vi "PSVCH_Demo_View.vi"() -> ()   [LabVIEW 2016]
panel:
  in  "Parameter":cluster{"Tag[]":string[], "Time":i64}={"Tag[]"=["VCH1"], "Time"=0}
  out "PData":waveform(dbl)[](graph)=[{"t0"=timestamp(3468473151.3644843 s since 1904-01-01), "dt"=0.001, "Y"=[6.739850074752029e-05, -0.00025439845700241445, -9.34999781361974e-05, -0.00025439845700241445, -0.00025439845700241445, -0.00025439845700241445, -0.0004152969358511465, -0.00025439845700241445, -0.00025439845700241445, 6.739850074752029e-05, -9.34999781361974e-05, -9.34999781361974e-05, -0.0004152969358511465, -9.34999781361974e-05, -0.0004152969358511465, 6.739850074752029e-05, -0.00025439845700241445, -0.00025439845700241445, 6.739850074752029e-05, -0.00025439845700241445, -9.34999781361974e-05, 0.00022829697964875422, -0.00025439845700241445, 0.00022829697964875422, 6.739850074752029e-05, 6.739850074752029e-05, -0.00025439845700241445, -0.00025439845700241445, -0.00025439845700241445, -9.34999781361974e-05, -9.34999781361974e-05, 6.739850074752029e-05, -0.00025439845700241445, -9.34999781361974e-05, -0.0004152969358511465, -0.00025439845700241445, 6.739850074752029e-05, -9.34999781361974e-05, -0.00025439845700241445, -0.00025439845700241445, -9.34999781361974e-05, 6.739850074752029e-05, 6.739850074752029e-05, 6.739850074752029e-05, -0.00025439845700241445, 0.00022829697964875422, -0.00025439845700241445, -0.0004152969358511465, -0.00025439845700241445, -9.34999781361974e-05], "attributes"=variant("NI_ChannelName"=variant(string "1"), "NI_UnitDescription"=variant(string "Volts"))}, {"t0"=timestamp(3468473151.364507 s since 1904-01-01), "dt"=0.001, "Y"=[-0.012665767574885531, -0.012665767574885531, -0.012826630906157108, -0.012826630906157108, -0.012826630906157108, -0.012826630906157108, -0.012504904243597582, -0.012665767574885531, -0.012665767574885531, -0.012665767574885531, -0.0131483575686512, -0.012504904243597582, -0.012665767574885531, -0.012826630906157108, -0.012826630906157108, -0.012826630906157108, -0.012826630906157108, -0.012987494237412326, -0.012665767574885531, -0.012826630906157108, -0.012987494237412326, -0.012504904243597582, -0.012826630906157108, -0.012826630906157108, -0.012826630906157108, -0.012826630906157108, -0.012987494237412326, -0.012665767574885531, -0.012987494237412326, -0.012987494237412326, -0.012826630906157108, -0.012826630906157108, -0.012826630906157108, -0.012826630906157108, -0.012665767574885531, -0.012826630906157108, -0.012826630906157108, -0.012826630906157108, -0.012665767574885531, -0.012504904243597582, -0.012826630906157108, -0.012504904243597582, -0.012987494237412326, -0.012826630906157108, -0.012826630906157108, -0.012826630906157108, -0.012826630906157108, -0.012826630906157108, -0.012826630906157108, -0.012987494237412326], "attributes"=variant("NI_ChannelName"=variant(string "2"), "NI_UnitDescription"=variant(string "Volts"))}, {"t0"=timestamp(3468473151.36453 s since 1904-01-01), "dt"=0.001, "Y"=[0.00011638367757987423, 0.00011638367757987423, 0.00027723671651823503, -4.446936134091291e-05, 0.00011638367757987423, 0.00011638367757987423, -4.446936134091291e-05, 0.0004380897554741851, -4.446936134091291e-05, -0.000205322400244142, -4.446936134091291e-05, 0.00027723671651823503, -4.446936134091291e-05, -4.446936134091291e-05, 0.00027723671651823503, 0.00027723671651823503, -4.446936134091291e-05, -4.446936134091291e-05, 0.00027723671651823503, -4.446936134091291e-05, 0.00027723671651823503, 0.00011638367757987423, -4.446936134091291e-05, 0.0004380897554741851, -4.446936134091291e-05, 0.00011638367757987423, 0.00011638367757987423, 0.00027723671651823503, 0.00011638367757987423, -4.446936134091291e-05, 0.00011638367757987423, 0.00011638367757987423, -4.446936134091291e-05, 0.00011638367757987423, -4.446936134091291e-05, -4.446936134091291e-05, -4.446936134091291e-05, -4.446936134091291e-05, 0.00011638367757987423, 0.00027723671651823503, 0.00011638367757987423, 0.00011638367757987423, -4.446936134091291e-05, 0.00011638367757987423, 0.00011638367757987423, 0.00027723671651823503, 0.00027723671651823503, 0.00027723671651823503, 0.00011638367757987423, -4.446936134091291e-05], "attributes"=variant("NI_ChannelName"=variant(string "3"), "NI_UnitDescription"=variant(string "Volts"))}, {"t0"=timestamp(3468473151.364553 s since 1904-01-01), "dt"=0.001, "Y"=[-0.01584889046687111, -0.01584889046687111, -0.01552708791201146, -0.015687989189449317, -0.015687989189449317, -0.01552708791201146, -0.016009791744276847, -0.015687989189449317, -0.01584889046687111, -0.01584889046687111, -0.01584889046687111, -0.016009791744276847, -0.01584889046687111, -0.016009791744276847, -0.015687989189449317, -0.01584889046687111, -0.016009791744276847, -0.01584889046687111, -0.01584889046687111, -0.015687989189449317, -0.015687989189449317, -0.015687989189449317, -0.01584889046687111, -0.01584889046687111, -0.015687989189449317, -0.01584889046687111, -0.015687989189449317, -0.01584889046687111, -0.01584889046687111, -0.016009791744276847, -0.015687989189449317, -0.01552708791201146, -0.015687989189449317, -0.015687989189449317, -0.01584889046687111, -0.015687989189449317, -0.015687989189449317, -0.015687989189449317, -0.01552708791201146, -0.016009791744276847, -0.015687989189449317, -0.015687989189449317, -0.01536618663455752, -0.01584889046687111, -0.016009791744276847, -0.016170693021666554, -0.015687989189449317, -0.015687989189449317, -0.01552708791201146, -0.01584889046687111], "attributes"=variant("NI_ChannelName"=variant(string "4"), "NI_UnitDescription"=variant(string "Volts"))}, {"t0"=timestamp(3468473151.364576 s since 1904-01-01), "dt"=0.001, "Y"=[0.005178231424439744, 0.005178231424439744, 0.005017342955467275, 0.005178231424439744, 0.005017342955467275, 0.005017342955467275, 0.005017342955467275, 0.005339119893430259, 0.005017342955467275, 0.005178231424439744, 0.005017342955467275, 0.005017342955467275, 0.005178231424439744, 0.005017342955467275, 0.005178231424439744, 0.005017342955467275, 0.005017342955467275, 0.005178231424439744, 0.004856454486512835, 0.005178231424439744, 0.004856454486512835, 0.005178231424439744, 0.005178231424439744, 0.005017342955467275, 0.005178231424439744, 0.005339119893430259, 0.005178231424439744, 0.005339119893430259, 0.005017342955467275, 0.005178231424439744, 0.005017342955467275, 0.005017342955467275, 0.005178231424439744, 0.005017342955467275, 0.005178231424439744, 0.005017342955467275, 0.005017342955467275, 0.005178231424439744, 0.005017342955467275, 0.005017342955467275, 0.005017342955467275, 0.005178231424439744, 0.005178231424439744, 0.005017342955467275, 0.004856454486512835, 0.005178231424439744, 0.005017342955467275, 0.005017342955467275, 0.005017342955467275, 0.005339119893430259], "attributes"=variant("NI_ChannelName"=variant(string "5"), "NI_UnitDescription"=variant(string "Volts"))}, {"t0"=timestamp(3468473151.364599 s since 1904-01-01), "dt"=0.001, "Y"=[-0.0034799763219972627, -0.003158190334419984, -0.0034799763219972627, -0.003319083328217264, -0.003319083328217264, -0.003319083328217264, -0.0034799763219972627, -0.003319083328217264, -0.0034799763219972627, -0.0034799763219972627, -0.0034799763219972627, -0.003319083328217264, -0.0034799763219972627, -0.003319083328217264, -0.003319083328217264, -0.0034799763219972627, -0.0036408693157599955, -0.0036408693157599955, -0.0034799763219972627, -0.0036408693157599955, -0.003158190334419984, -0.002997297340605406, -0.003319083328217264, -0.0034799763219972627, -0.0034799763219972627, -0.0034799763219972627, -0.0034799763219972627, -0.0036408693157599955, -0.003319083328217264, -0.0036408693157599955, -0.0034799763219972627, -0.0036408693157599955, -0.003319083328217264, -0.003319083328217264, -0.003158190334419984, -0.003319083328217264, -0.003319083328217264, -0.003319083328217264, -0.003319083328217264, -0.003319083328217264, -0.003158190334419984, -0.0034799763219972627, -0.0036408693157599955, -0.0036408693157599955, -0.003158190334419984, -0.0034799763219972627, -0.003319083328217264, -0.003319083328217264, -0.0034799763219972627, -0.0034799763219972627], "attributes"=variant("NI_ChannelName"=variant(string "6"), "NI_UnitDescription"=variant(string "Volts"))}, {"t0"=timestamp(3468473151.364622 s since 1904-01-01), "dt"=0.001, "Y"=[-0.0043366992498497115, -0.004014895158054102, -0.004175797203960548, -0.004175797203960548, -0.004014895158054102, -0.004014895158054102, -0.004175797203960548, -0.004014895158054102, -0.0043366992498497115, -0.004014895158054102, -0.004014895158054102, -0.0043366992498497115, -0.0043366992498497115, -0.0043366992498497115, -0.004014895158054102, -0.004175797203960548, -0.004014895158054102, -0.004497601295721608, -0.004175797203960548, -0.004497601295721608, -0.004014895158054102, -0.004014895158054102, -0.004658503341576253, -0.0043366992498497115, -0.004175797203960548, -0.0043366992498497115, -0.0043366992498497115, -0.004175797203960548, -0.0043366992498497115, -0.0043366992498497115, -0.004014895158054102, -0.004014895158054102, -0.004175797203960548, -0.004175797203960548, -0.004497601295721608, -0.004014895158054102, -0.004175797203960548, -0.004175797203960548, -0.0043366992498497115, -0.0043366992498497115, -0.004014895158054102, -0.004175797203960548, -0.0043366992498497115, -0.004175797203960548, -0.0043366992498497115, -0.004175797203960548, -0.004014895158054102, -0.004014895158054102, -0.004175797203960548, -0.004014895158054102], "attributes"=variant("NI_ChannelName"=variant(string "7"), "NI_UnitDescription"=variant(string "Volts"))}, {"t0"=timestamp(3468473151.364645 s since 1904-01-01), "dt"=0.001, "Y"=[-0.004637349833195447, -0.004637349833195447, -0.004637349833195447, -0.0044764991715924955, -0.0047982004947813555, -0.0044764991715924955, -0.0047982004947813555, -0.0047982004947813555, -0.004637349833195447, -0.0044764991715924955, -0.004637349833195447, -0.0044764991715924955, -0.0049590511563502365, -0.0047982004947813555, -0.004637349833195447, -0.004637349833195447, -0.0047982004947813555, -0.004637349833195447, -0.0047982004947813555, -0.004637349833195447, -0.0049590511563502365, -0.0047982004947813555, -0.0047982004947813555, -0.004637349833195447, -0.004637349833195447, -0.004637349833195447, -0.004637349833195447, -0.0044764991715924955, -0.0044764991715924955, -0.0049590511563502365, -0.0047982004947813555, -0.004637349833195447, -0.004637349833195447, -0.0044764991715924955, -0.004637349833195447, -0.004637349833195447, -0.0044764991715924955, -0.004637349833195447, -0.004637349833195447, -0.004637349833195447, -0.004315648509972485, -0.0047982004947813555, -0.004637349833195447, -0.004637349833195447, -0.004637349833195447, -0.004637349833195447, -0.0047982004947813555, -0.004637349833195447, -0.0047982004947813555, -0.0047982004947813555], "attributes"=variant("NI_ChannelName"=variant(string "8"), "NI_UnitDescription"=variant(string "Volts"))}] caption="虚拟通道波形"
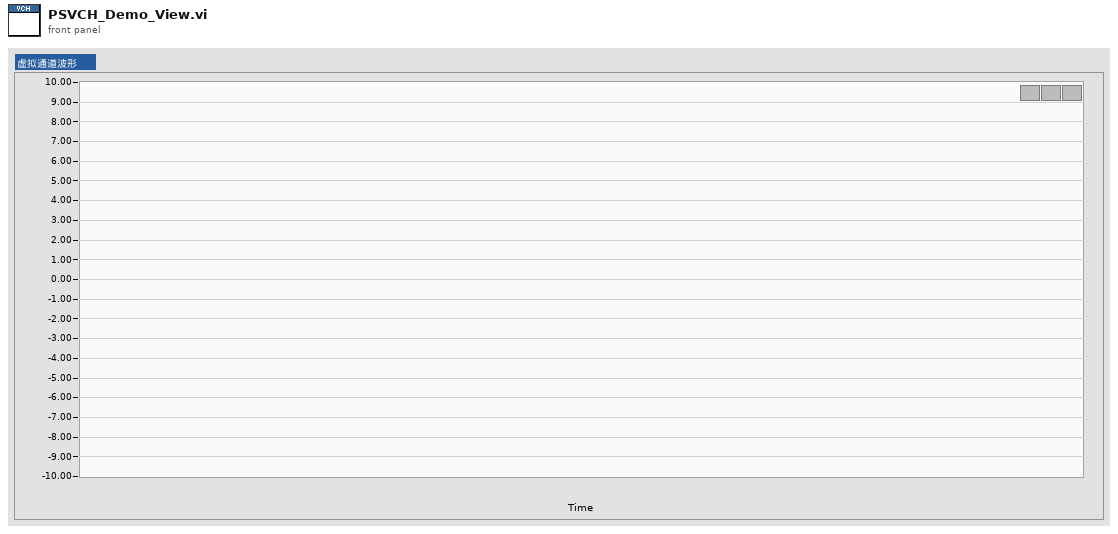
[diagram p1: front panel]
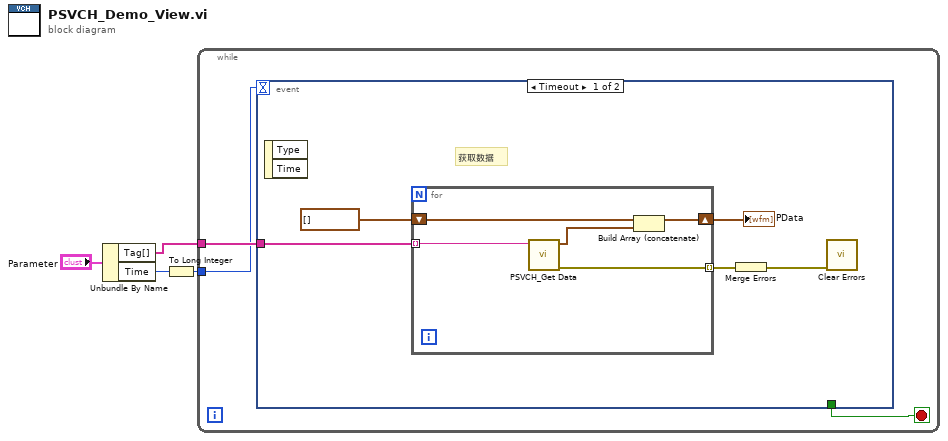
[diagram p0: block diagram]
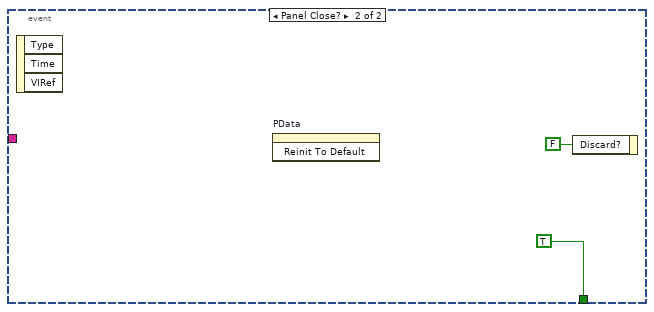
[diagram p2: hidden frame]
diagram:
  n1 = Unbundle By Name("Parameter") -> ("Tag[]"=w3:string[], "Time"=w2:i64)
  n2 = To Long Integer(number=w2) -> (32bit integer=w1:i32)
  n3 = while {
    tunnel: w3 -> [w6]
    tunnel: w1 -> [w5]
    stop <- w7 stop-if-true
    n4 = event shown="[0] Timeout" {
      selector: _ -> [_ _]
      dyn-events: _ -> [_ _]
      timeout: w5 -> [_ _]
      tunnel: [_ TRUE ("放弃？")] -> w7
      tunnel: w6 -> [w12 _]
      event Timeout {
        # "获取数据"
        n5 = event-data() -> ()  [unwired: 1 in, 2 out]
        n6 = for {
          tunnel: w12 -> [w17] mode=indexing
          shift-right: [w14] -> w10
          shift-left: waveform(dbl)[] [] ("Out") -> [w15]
          tunnel: [w13] -> w8 mode=indexing
          n7 = call "PSVCH_Get Data.vi"("ChlName"=w17) -> ("Error Out"=w13:errorcluster, "Data"=w16:waveform(dbl))  [unwired: 8 in, 1 out]
          n8 = Build Array (concatenate)(w15, w16) -> (w14:waveform(dbl)[])
        }
        "PData" <- w10
        n9 = Merge Errors(w8) -> (w9:errorcluster)
        n10 = call <vilib>:"Clear Errors.vi"("error in (no error)"=w9) -> ()  [unwired: 5 in, 2 out]
      }
      event Panel Close? {
        n11 = event-data() -> ()  [unwired: 1 in, 3 out]
        n12 = invoke on="PData" class="WFChart (严格)" method="Reinit To Default"() -> ()  [unwired: 3 in, 3 out]
        n13 = event-data("Discard?"=FALSE ("放弃？")) -> ()  [unwired: 1 in, 1 out]
      }
    }
  }
